vi "Execute-RT-Deploy.vi"   [LabVIEW 2014]
uses:
  <vilib>/Utility/error.llb/DialogType.ctl
  <vilib>/Wiresmith Technology/LabVIEW CLI/CLI Class/CLI.lvclass
types:
  T1 = cluster{"time to run VI":u32, "time to start VI":u32}
  T2 = typedef "DialogType.ctl" = u16
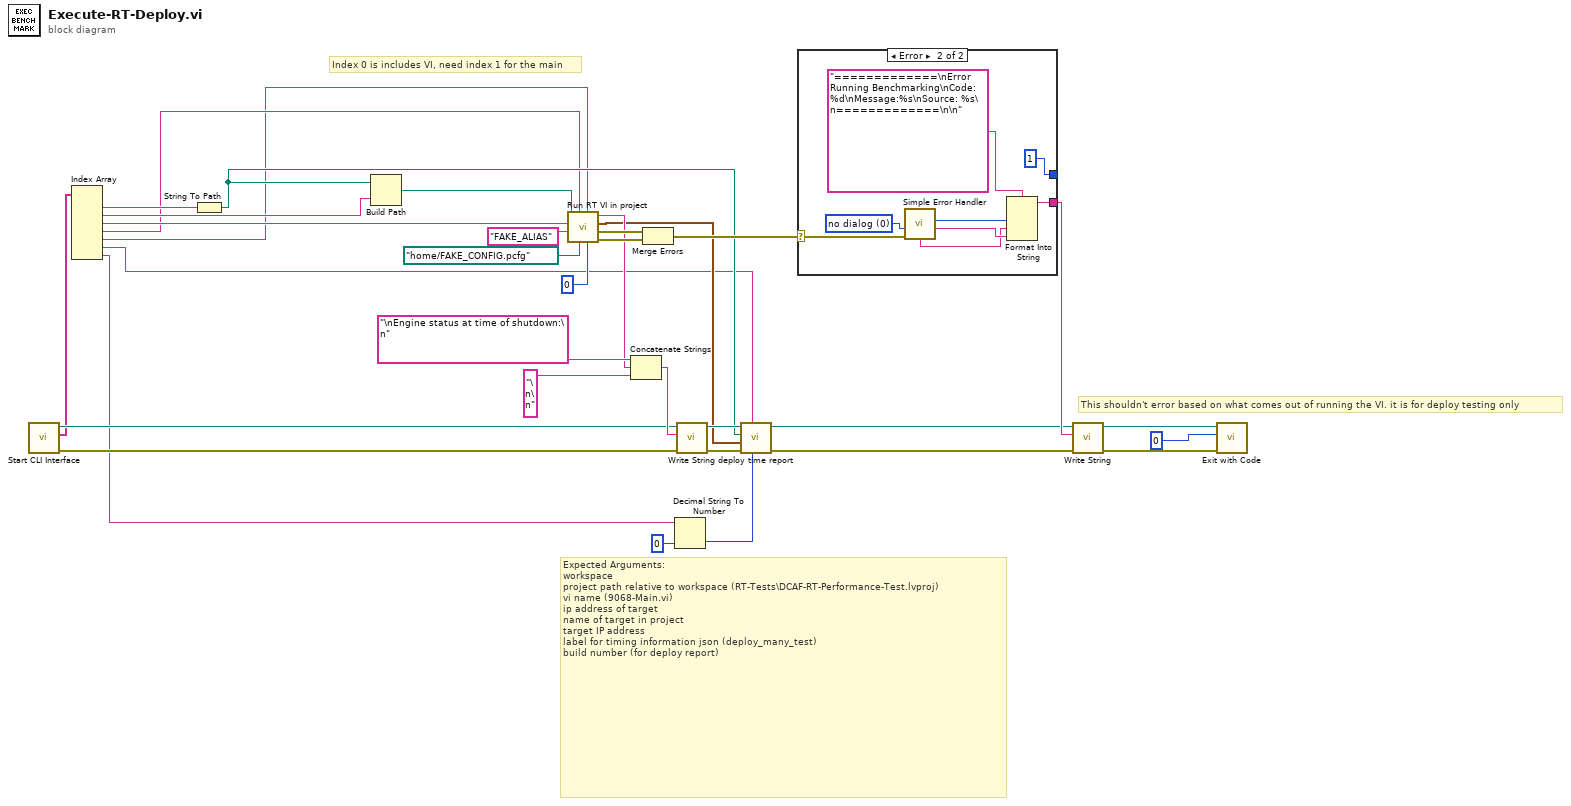
[diagram p0: block diagram]
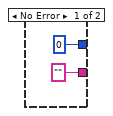
[diagram p2: hidden frame]
diagram:
  # "This shouldn't error based on what comes out of running the VI. it is for deploy testing only"
  # "Expected Arguments:\nworkspace \nproject path relative to workspace (RT-Tests\\DCAF-RT-Performance-Test.lvproj)\nvi name (9068-Main.vi)\nip address of target\nname of target in project\ntarget IP address\nlabel for timing information json (deploy_many_test)\nbuild number (for deploy report)"
  # "Index 0 is includes VI, need index 1 for the main"
  n1 = call <vilib>:"Start CLI Interface.vi"() -> ("error out"=w25:errorcluster, "Custom Parameters"=w6:string[], "CLI out"=w26:refnum<class "CLI.lvclass">)  [unwired: 9 in]
  n2 = Index Array(array=w6) -> (element #1=w9:string, element #2=w8:string, element #3=w7:string, element #4=w5:string, element #5=w4:string, element #6=w3:string, element #7=w1:string)  [unwired: 7 in]
  n3 = String To Path(string=w9) -> (path=w16:path)
  n4 = Build Path(base path=w16, name or relative path=w8) -> (appended path=w31:path)
  n5 = call "Run RT VI in project.vi"("Run Time"=u32 0, "project target"=w4, "configuration file path"=path "/home/FAKE_CONFIG.pcfg", "ip address"=w5, "target alias"="FAKE_ALIAS", "vi name"=w7, "Project Path"=w31) -> ("error out"=w30:errorcluster, "invoked VI error out"=w29:errorcluster, "timing"=w17:T1, "engine status"=w22:string)  [unwired: 1 in]
  n6 = Concatenate Strings("\nEngine status at time of shutdown:\n" ("string"), w22, "\n\n" ("string")) -> (w27:string)
  n7 = Merge Errors(w29, w30) -> (w28:errorcluster)
  n8 = Decimal String To Number(string=w1, default (0L)=u32 0 ("default (0 I32)")) -> (number=w14:u32)  [unwired: 1 in, 1 out]
  n9 = call <vilib>:"Write String.vi"("error in (no error)"=w25, "Text to Write"=w27, "CLI in"=w26) -> ("error out"=w19:errorcluster, "CLI out"=w21:refnum<class "CLI.lvclass">)  [unwired: 7 in]
  n10 = call "deploy time report.vi"("build_number"=w14, "test name"=w3, "error in (no error)"=w19, "timing"=w17, "workspace path"=w16, "CLI in"=w21) -> ("error out"=w18:errorcluster, "CLI out"=w20:refnum<class "CLI.lvclass">)  [unwired: 4 in]
  n11 = case shown="Error" w28 {
    selector: w28 -> [_ w40]
    tunnel: ["" w36] -> w32
    tunnel: [0 ("Exit Code (0)") 1 ("Exit Code (0)")] -> _
    frame No Error {
    }
    frame Error {
      w41 = T2 0 items=["no dialog", "OK message", "continue or stop message", "OK message + warnings", "continue/stop + warnings"] ("type of dialog (OK msg:1)")
      n12 = call <vilib>:"Simple Error Handler.vi"("type of dialog (OK msg:1)"=w41, "error in (no error)"=w40) -> ("code out"=w39:i32, "source out"=w38:string, "message"=w37:string)  [unwired: 3 in, 2 out]
      n13 = Format Into String(format string="=============\nError Running Benchmarking\nCode: %d\nMessage:%s\nSource: %s\n=============\n\n", w39, w37, w38) -> (resulting string=w36:string)  [unwired: 2 in, 1 out]
    }
  }
  n14 = call <vilib>:"Write String.vi"("error in (no error)"=w18, "Text to Write"=w32, "CLI in"=w20) -> ("error out"=w15:errorcluster, "CLI out"=w33:refnum<class "CLI.lvclass">)  [unwired: 7 in]
  n15 = call <vilib>:"Exit with Code.vi"("error in (no error)"=w15, "Exit Code (0)"=0 ("t"), "CLI in"=w33) -> ()  [unwired: 8 in, 1 out]
